vi "Read Local OOB Data.vi"(8 "error in":errorcluster, 11 "OOB in":refnum<class "CIFOutOfBand.lvclass">) -> (0 "error out":errorcluster, 2 "Local OOB Data":variant, 3 "OOB out":refnum<class "CIFOutOfBand.lvclass">)   [LabVIEW 2021, in "CIFOutOfBand.lvclass"]
uses:
  CIFOutOfBand.lvclass
  CIFOutOfBand.lvclass/CIFOutOfBand.ctl
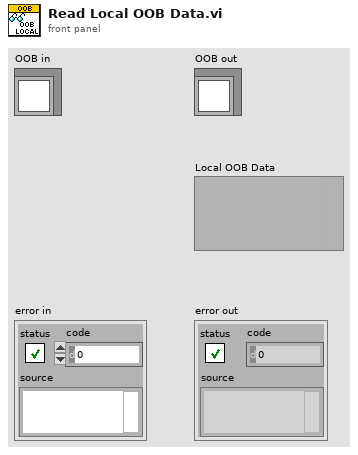
[diagram p1: front panel]
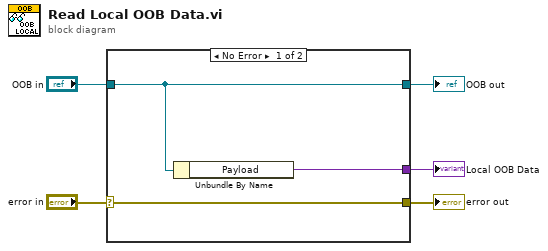
[diagram p0: block diagram]
diagram:
  n1 = case shown="No Error" "error in" {
    selector: "error in" -> [w8 w9]
    tunnel: [w8 w9] -> w4
    tunnel: [w7 w10] -> w2
    tunnel: "OOB in" -> [w7 w10]
    tunnel: [w6 _] -> w1
    frame No Error {
      n2 = Unbundle By Name(w7) -> ("Payload"=w6:variant)
    }
    frame Error {
    }
  }
  "error out" <- w4
  "OOB out" <- w2
  "Local OOB Data" <- w1
